vi "initialize FPGA Custom Device.vi"(8 "error in (no error)":errorcluster, 11 "Item Ref in":T1 format="%.0x") -> (0 "error out":errorcluster, 3 "Item Ref out":T1 format="%.0x")   [LabVIEW 2016, in "FPGA Resource Manager System Defintion.lvlib"]
uses:
  FPGA Resource Manager System Defintion.lvlib
  <vilib>/NI Veristand/Custom Device API/Custom Device Item Ref.ctl
  global constants.vi
  <vilib>/NI Veristand/Custom Device API/Custom Device API.lvlib
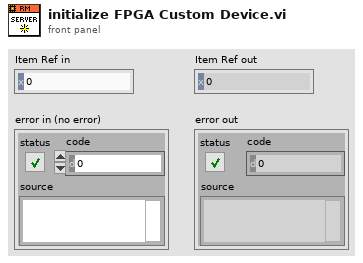
[diagram p1: front panel]
types:
  T1 = typedef "Custom Device API.lvlib/Custom Device Item Ref.ctl" = u64
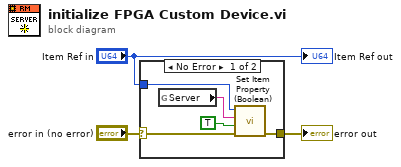
[diagram p0: block diagram]
diagram:
  n1 = case shown="No Error" "error in (no error)" {
    selector: "error in (no error)" -> [w8 w9]
    tunnel: [w7 w9] -> w2
    tunnel: "Item Ref in" -> [w6 _]
    frame No Error {
      n2 = global read "global constants.vi" "Server"() -> (w5:string)
      n3 = call <vilib>:"Set Item Property (Boolean).vi"("error in (no error)"=w8, "Value"=TRUE, "Property Name"=w5, "Item Ref in"=w6) -> ("error out"=w7:errorcluster)  [unwired: 5 in, 2 out]
    }
    frame Error {
    }
  }
  "error out" <- w2
  "Item Ref out" <- "Item Ref in"
